vi "Rect (SubVI).vi"(11 "dimensions (w,h)":T1) -> (3 "Cluster":cluster{"x":i16, "y":i16, u32, u32})   [LabVIEW 2019]
uses:
  <vilib>/Utility/miscctls.llb/LVBoundsTypeDef.ctl
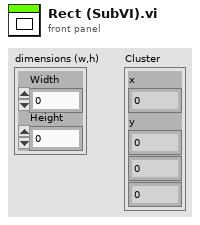
[diagram p1: front panel]
types:
  T1 = typedef "LVBoundsTypeDef.ctl" = cluster{"Width":u32, "Height":u32}
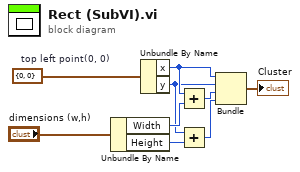
[diagram p0: block diagram]
diagram:
  w1 = cluster{"x":i16, "y":i16} {"x"=0, "y"=0}  # top left point(0, 0)
  n1 = Unbundle By Name("dimensions (w,h)") -> ("Width"=w7:u32, "Height"=w6:u32)
  n2 = Unbundle By Name(w1) -> ("x"=w5:i16, "y"=w4:i16)
  n3 = Add(x=w5, y=w7) -> (x+y=w3:u32)
  n4 = Add(x=w4, y=w6) -> (x+y=w2:u32)
  n5 = Bundle("x"=w5, "y"=w4, w3, w2) -> (→"Cluster":cluster{"x":i16, "y":i16, u32, u32})  [unwired: 1 in]
